vi "User Console View.vi"(8 "error in (no error)":errorcluster, 11 "View Model":T1) -> (0 "error out":errorcluster)   [LabVIEW 2017]
doc: "This simulated HW Console View. Contains human input."
uses:
  View Model/Controls/View Model.ctl
  Error Handler/Controls/Error Model.ctl
  Error Handler/Controls/Error Type.ctl
  View Model/Controls/Shared Model.ctl
  Elevator Controller/Controls/Elevator Model.ctl
  Elevator Controller/Controls/Controller Overhead.ctl
  Elevator Controller/Controls/Elevator Commands.ctl
  Configuration/Controls/Configuration Model.ctl
  Configuration/Controls/Configuration Data.ctl
  Controls/User Console View.ctl
panel:
  in  "Emergency":bool
  in  "Close Door":bool
  in  "Open Door":bool
  in  "1st Floor":bool
  in  "2nd Floor":bool
  in  "3rd Floor":bool
  in  "4th Floor":bool
  in  "Up 1":bool
  in  "Up 2":bool
  in  "Up 3":bool
  in  "Down 2":bool
  in  "Down 3":bool
  in  "Down 4":bool
  # "[Covers: UI1]"
  # "Elevator Call"
  # "Floor Selection"
  # "[Covers UI2A1]"
  # "Door Buttons"
  # "[Covers: UI2C]"
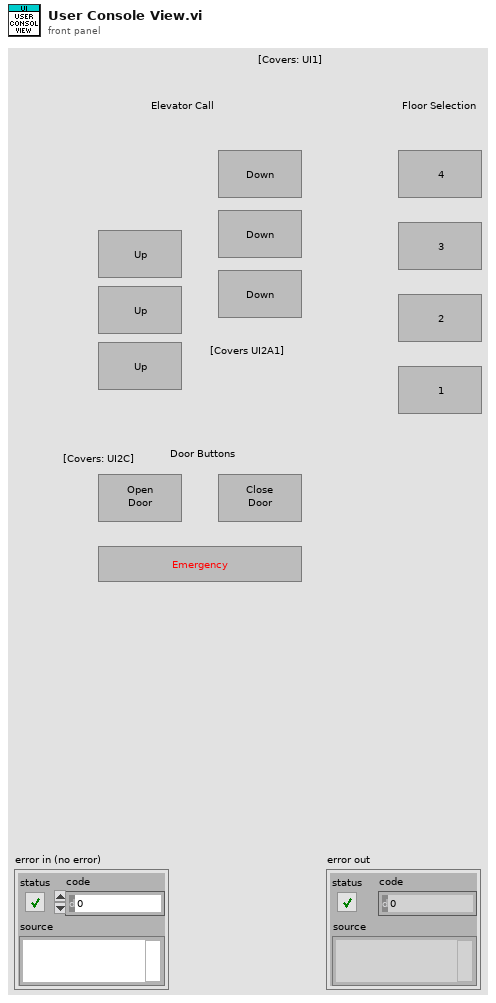
[diagram p1: front panel]
types:
  T1 = typedef "View Model.ctl" = cluster{"Error Model":T2, "Shared Model":T3, "Elevator Model":T4, "Configuration Model":T5}
  T2 = typedef "Error Model.ctl" = cluster{"Error Event":refnum<user-event>}
  T3 = typedef "Shared Model.ctl" = cluster{"Stop DVR":refnum<data-value>, "Stop Event":refnum<user-event>}
  T4 = typedef "Elevator Model.ctl" = cluster{"Controller Overhead":refnum<data-value>, "Motion Change":refnum<user-event>, "Direction Change":refnum<user-event>, "Door Position Change":refnum<user-event>, "Emergency Change":refnum<user-event>, "Floor Change":refnum<user-event>, "Elevator Cmd":refnum<user-event>}
  T5 = typedef "Configuration Model.ctl" = cluster{"Configuration":refnum<data-value>, "Config Change":refnum<user-event>}
  T6 = typedef "User Console View.ctl" = cluster{"Down 2":refnum<vi>, "Down 3":refnum<vi>, "Down 4":refnum<vi>, "Up 1":refnum<vi>, "Up 2":refnum<vi>, "Up 3":refnum<vi>, "1st Floor":refnum<vi>, "2nd Floor":refnum<vi>, "3rd Floor":refnum<vi>, "4th Floor":refnum<vi>, "Open Door":refnum<vi>, "Close Door":refnum<vi>, "Emergency":refnum<vi>}
  T7 = typedef "Elevator Commands.ctl" = enum16{"Go Up", "Go Down", "Go To Floor", "Emergency", "Open Doors", "Close Doors"}
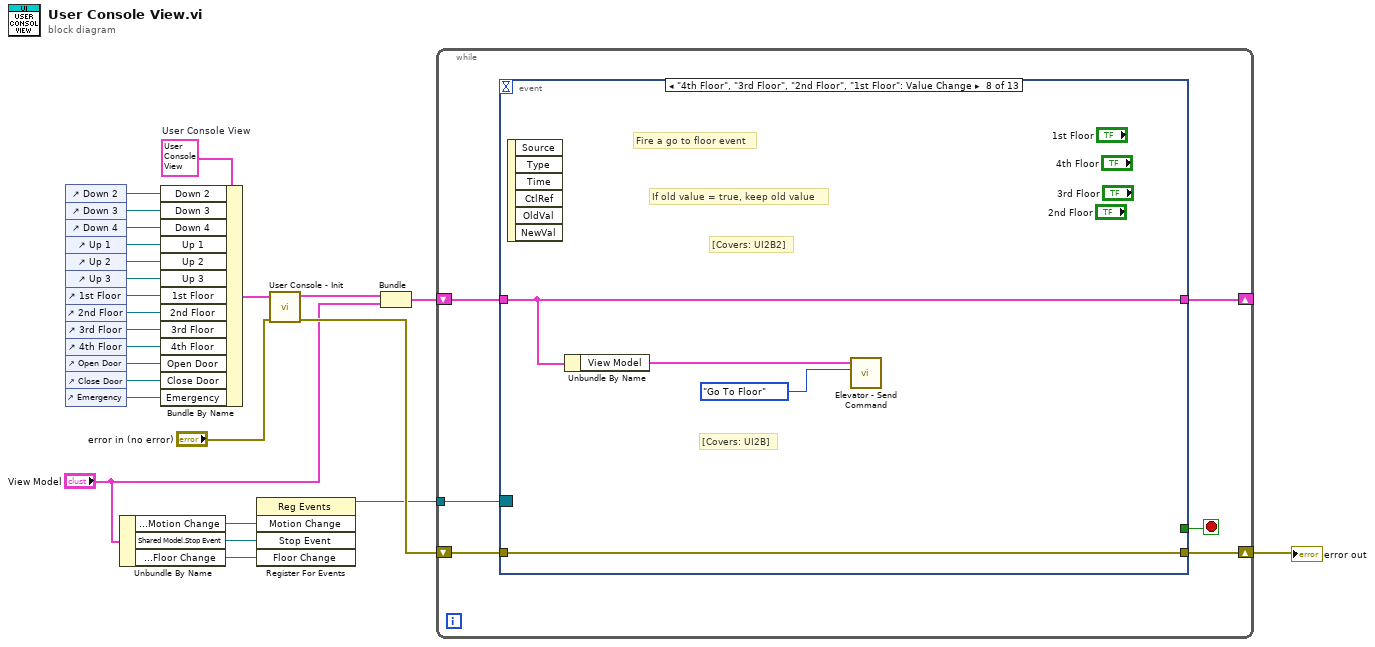
[diagram p0: block diagram]
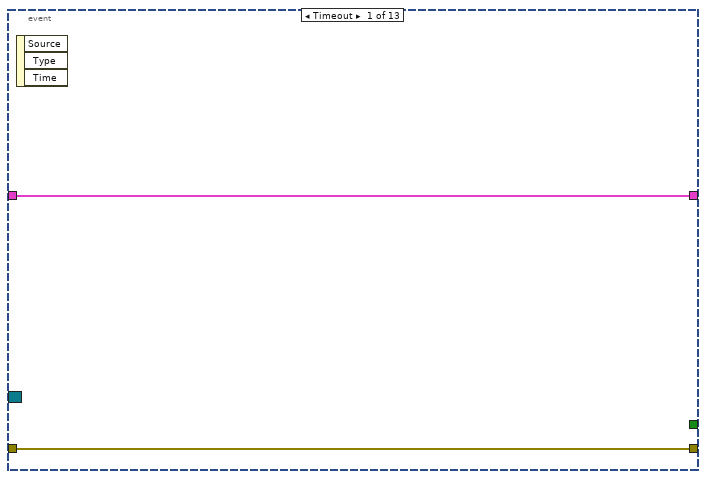
[diagram p2: hidden frame]
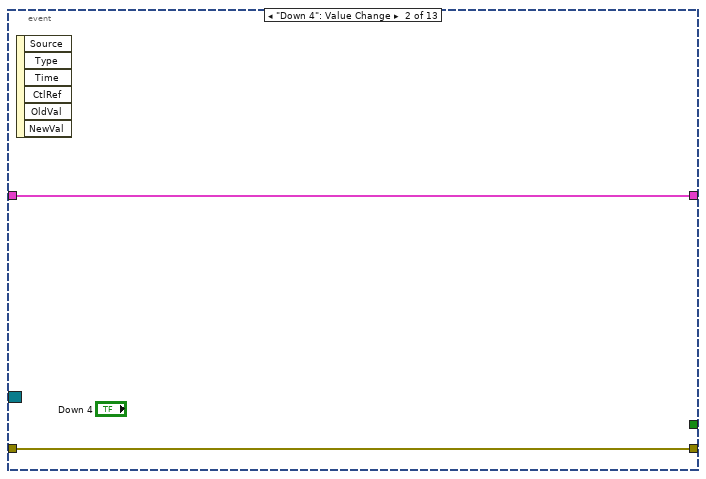
[diagram p3: hidden frame]
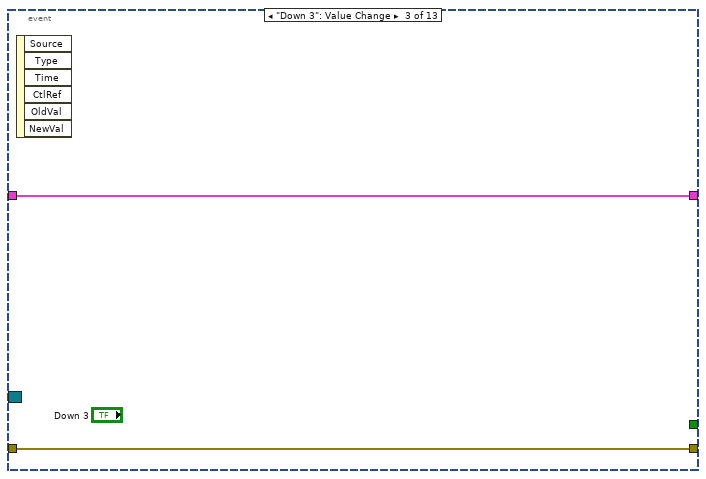
[diagram p4: hidden frame]
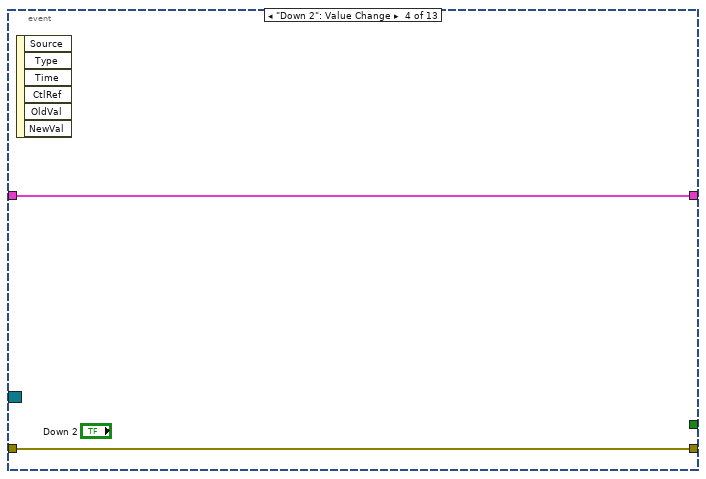
[diagram p5: hidden frame]
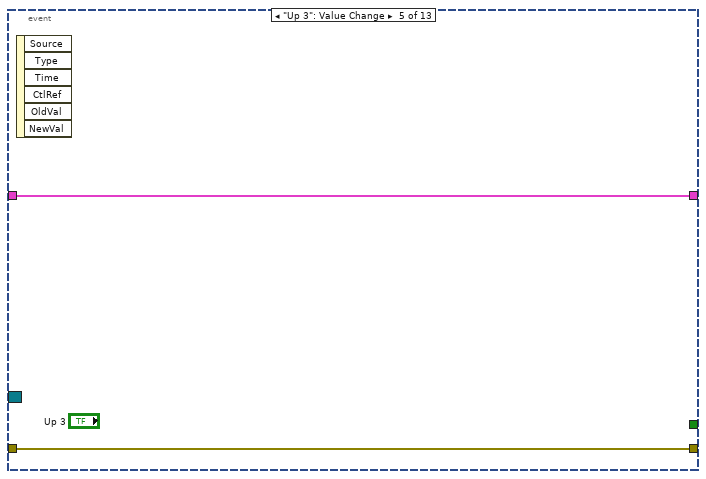
[diagram p6: hidden frame]
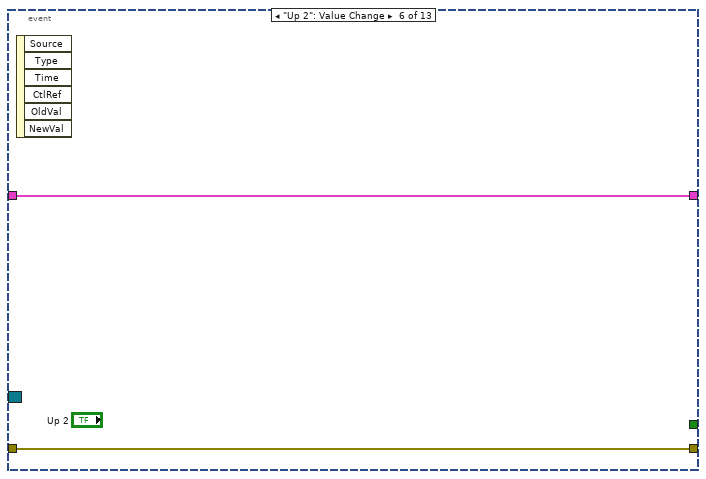
[diagram p7: hidden frame]
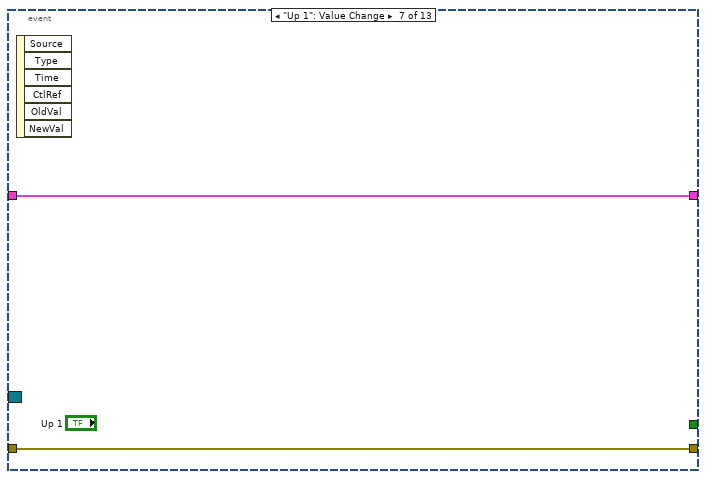
[diagram p8: hidden frame]
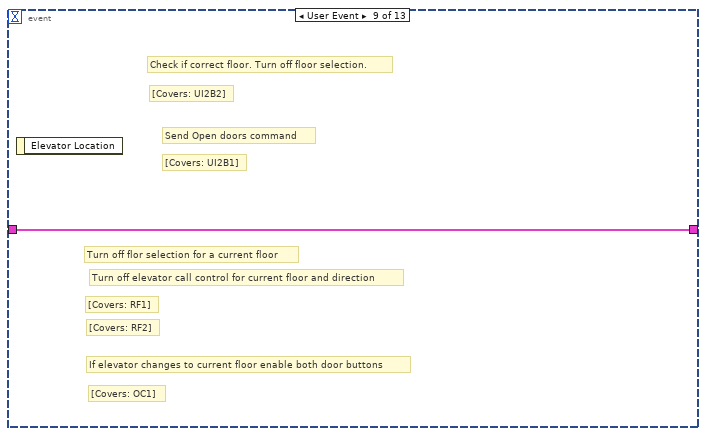
[diagram p9: hidden frame]
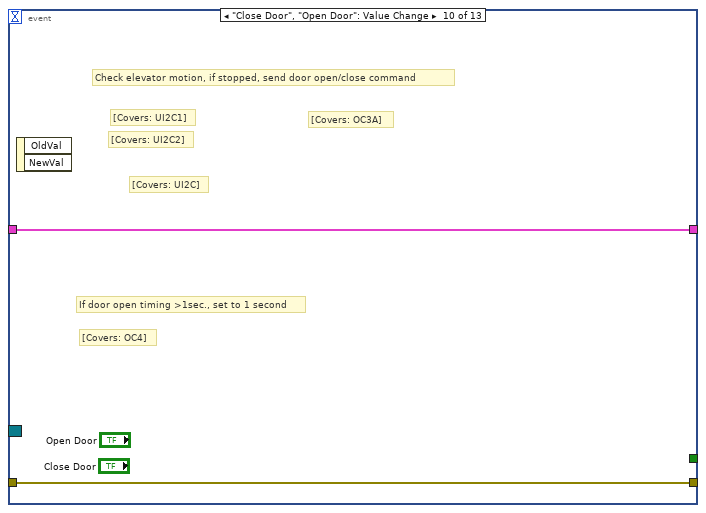
[diagram p10: hidden frame]
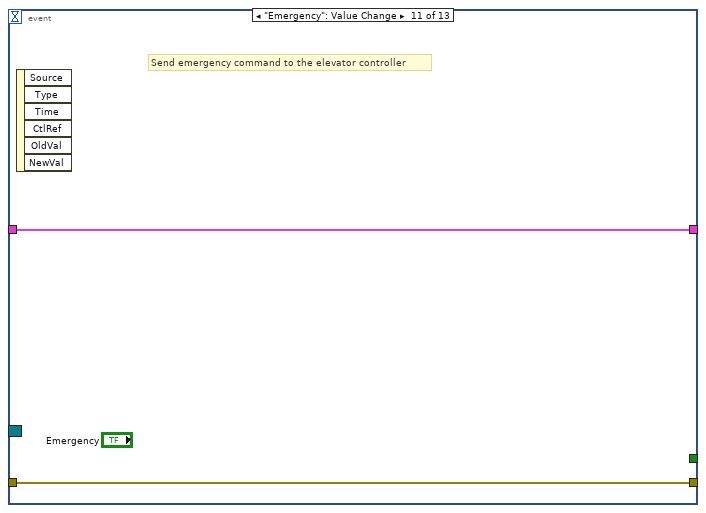
[diagram p11: hidden frame]
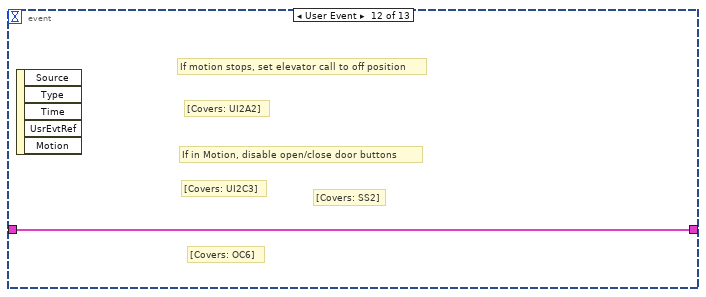
[diagram p12: hidden frame]
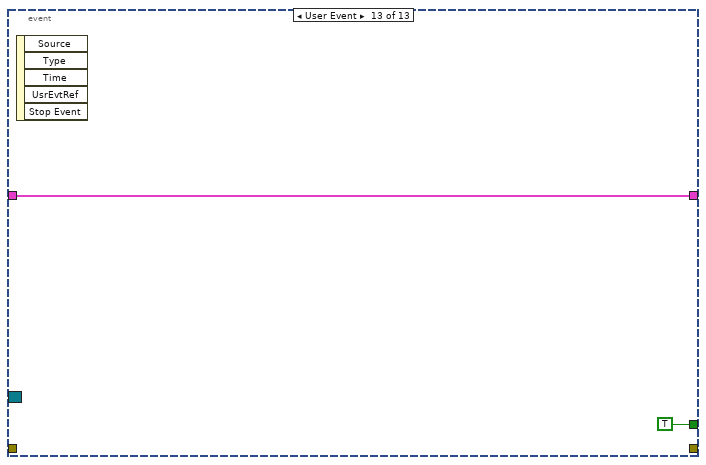
[diagram p13: hidden frame]
diagram:
  w12 = T6 {"Down 2"=refnum, "Down 3"=refnum, "Down 4"=refnum, "Up 1"=refnum, "Up 2"=refnum, "Up 3"=refnum, "1st Floor"=refnum, "2nd Floor"=refnum, "3rd Floor"=refnum, "4th Floor"=refnum, "Open Door"=refnum, "Close Door"=refnum, "Emergency"=refnum}  # User Console View
  n1 = control-ref of="Down 2"() -> (w25:refnum<vi>)
  n2 = control-ref of="Down 3"() -> (w24:refnum<vi>)
  n3 = control-ref of="Down 4"() -> (w23:refnum<vi>)
  n4 = control-ref of="Up 1"() -> (w22:refnum<vi>)
  n5 = control-ref of="Up 2"() -> (w21:refnum<vi>)
  n6 = control-ref of="Up 3"() -> (w20:refnum<vi>)
  n7 = control-ref of="1st Floor"() -> (w19:refnum<vi>)
  n8 = control-ref of="2nd Floor"() -> (w18:refnum<vi>)
  n9 = control-ref of="3rd Floor"() -> (w17:refnum<vi>)
  n10 = control-ref of="4th Floor"() -> (w16:refnum<vi>)
  n11 = control-ref of="Open Door"() -> (w15:refnum<vi>)
  n12 = control-ref of="Close Door"() -> (w14:refnum<vi>)
  n13 = control-ref of="Emergency"() -> (w13:refnum<vi>)
  n14 = Unbundle By Name("View Model") -> ("Elevator Model.Motion Change"=w4:refnum<user-event>, "Shared Model.Stop Event"=w2:refnum<user-event>, "Elevator Model.Floor Change"=w1:refnum<user-event>)
  n15 = Bundle By Name(cluster=w12, "Down 2"=w25, "Down 3"=w24, "Down 4"=w23, "Up 1"=w22, "Up 2"=w21, "Up 3"=w20, "1st Floor"=w19, "2nd Floor"=w18, "3rd Floor"=w17, "4th Floor"=w16, "Open Door"=w15, "Close Door"=w14, "Emergency"=w13) -> (w10:T6)
  n16 = register-events(w4, w2, w1) -> (reference out=w3:refnum<event-registration>)  [unwired: 2 in, 1 out]
  n17 = call "User Console - Init.vi"("error in (no error)"="error in (no error)", "User Console View"=w10) -> ("error out"=w8:errorcluster, "User Console View"=w7:T6)  [unwired: 8 in]
  n18 = Bundle("User Console View"=w7, "View Model"="View Model") -> (w6:cluster{"User Console View":T6, "View Model":T1})  [unwired: 1 in]
  n19 = while {
    shift-right: [w28] -> _
    shift-left: w6 -> [w31]
    shift-right: [w29] -> w11
    shift-left: w8 -> [w30]
    tunnel: w3 -> [w27]
    stop <- w26 stop-if-true
    n20 = event shown="[7] \"4th Floor\", \"3rd Floor\", \"2nd Floor\", \"1st Floor\": Value Change" {
      selector: w27 -> [_ _ _ _ _ _ _ _ _ _ _ _ _]
      dyn-events: _ -> [_ _ _ _ _ _ _ _ _ _ _ _ _]
      timeout: _ -> [_ _ _ _ _ _ _ _ _ _ _ _ _]
      tunnel: w31 -> [w32 w34 w36 w38 w40 w42 w44 w47 w50 w51 w53 w55 w57]
      tunnel: w30 -> [w33 w35 w37 w39 w41 w43 w45 w49 _ w52 w54 _ _]
      tunnel: [w33 w35 w37 w39 w41 w43 w45 w49 _ w52 w54 _ _] -> w29
      tunnel: [w32 w34 w36 w38 w40 w42 w44 w47 w50 w51 w53 w55 w57] -> w28
      tunnel: [_ _ _ _ _ _ _ _ _ _ _ _ TRUE] -> w26
      event Timeout {
        n21 = event-data() -> ()  [unwired: 1 in, 3 out]
      }
      event "Down 4": Value Change {
        n22 = event-data() -> ()  [unwired: 1 in, 6 out]
      }
      event "Down 3": Value Change {
        n23 = event-data() -> ()  [unwired: 1 in, 6 out]
      }
      event "Down 2": Value Change {
        n24 = event-data() -> ()  [unwired: 1 in, 6 out]
      }
      event "Up 3": Value Change {
        n25 = event-data() -> ()  [unwired: 1 in, 6 out]
      }
      event "Up 2": Value Change {
        n26 = event-data() -> ()  [unwired: 1 in, 6 out]
      }
      event "Up 1": Value Change {
        n27 = event-data() -> ()  [unwired: 1 in, 6 out]
      }
      event "4th Floor", "3rd Floor", "2nd Floor", "1st Floor": Value Change {
        # "[Covers: UI2B]"
        # "[Covers: UI2B2]"
        # "If old value = true, keep old value"
        # "Fire a go to floor event"
        n28 = event-data() -> ()  [unwired: 1 in, 6 out]
        n29 = Unbundle By Name(w47) -> ("View Model"=w48:T1)
        n30 = call "Elevator - Send Command.vi"("Elevator Commands"=Elevator_Commands."Go To Floor", "View Model"=w48) -> ()  [unwired: 8 in, 2 out]
      }
      event User Event {
        # "[Covers: OC1]"
        # "If elevator changes to current floor enable both door buttons"
        # "[Covers: RF2]"
        # "Turn off elevator call control for current floor and direction"
        # "[Covers: RF1]"
        # "Turn off flor selection for a current floor"
        # "[Covers: UI2B1]"
        # "Send Open doors command"
        # "Check if correct floor. Turn off floor selection."
        # "[Covers: UI2B2]"
        n31 = event-data() -> ()  [unwired: 1 in, 1 out]
      }
      event "Close Door", "Open Door": Value Change {
        # "[Covers: OC4]"
        # "If door open timing >1sec., set to 1 second"
        # "[Covers: OC3A]"
        # "[Covers: UI2C]"
        # "[Covers: UI2C2]"
        # "[Covers: UI2C1]"
        # "Check elevator motion, if stopped, send door open/close command"
        n32 = event-data() -> ()  [unwired: 1 in, 2 out]
      }
      event "Emergency": Value Change {
        # "Send emergency command to the elevator controller"
        n33 = event-data() -> ()  [unwired: 1 in, 6 out]
      }
      event User Event {
        # "[Covers: OC6]"
        # "[Covers: SS2]"
        # "[Covers: UI2C3]"
        # "If in Motion, disable open/close door buttons"
        # "[Covers: UI2A2]"
        # "If motion stops, set elevator call to off position"
        n34 = event-data() -> ()  [unwired: 1 in, 5 out]
      }
      event User Event {
        n35 = event-data() -> ()  [unwired: 1 in, 5 out]
      }
    }
  }
  "error out" <- w11
